vi "Nested Aliases.vi"(11 "Self Actor":refnum<class "Self Actor.lvclass">) -> (0 "error out":errorcluster, 2 "Nested Aliases":string[](array[string]))   [LabVIEW 2021, in "jettl.lvlib" / "Self Actor.lvclass"]
uses:
  Self Actor.lvclass
  Self Actor.lvclass/Self Actor.ctl
  jettl.lvlib
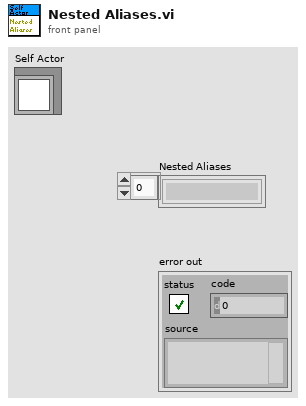
[diagram p1: front panel]
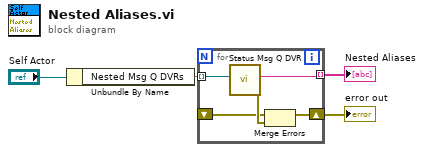
[diagram p0: block diagram]
diagram:
  n1 = Unbundle By Name("Self Actor") -> ("Nested Msg Q DVRs"=w1:set{refnum<data-value>})
  n2 = for {
    tunnel: w1 -> [w9] mode=indexing
    tunnel: [w8] -> w4 mode=indexing
    shift-right: [w6] -> w3
    shift-left: _ -> [w5]
    n3 = call "Status Msg Q DVR.vi"("Msg Q DVR"=w9) -> ("error out"=w7:errorcluster, "Msg Q DVR Alias"=w8:string)  [unwired: 9 in]
    n4 = Merge Errors(w5, w7) -> (w6:errorcluster)
  }
  "error out" <- w3
  "Nested Aliases" <- w4
